vi "DSF.Shared.Constants.vi"   [LabVIEW 2016, in "DSF.Shared.lvlib"]
uses:
  DSF.Shared.lvlib
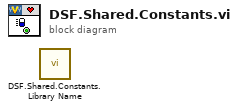
[diagram p0: block diagram]
diagram:
  n1 = call "DSF.Shared.Constants.Library Name.vi"() -> ()  [unwired: 11 in, 1 out]
